vi "Create-Destroy.vi"(8 "Error In":errorcluster) -> (0 "Error Out":errorcluster)   [LabVIEW 2017, in "Tests.lvlib"]
uses:
  Tests.lvlib
  <vilib>/addons/_JKI Toolkits/Caraya/classes/Test/Test.lvclass
  <vilib>/addons/_JKI Toolkits/Caraya/classes/Assert/Assert.lvclass
  src/LabSSH2/Public/Context/Context.lvclass
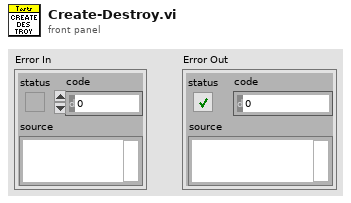
[diagram p1: front panel]
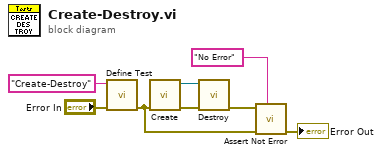
[diagram p0: block diagram]
diagram:
  n1 = call <vilib>:"Define Test.vi"("error in (no error)"="Error In", "Label (VI Title)"="Create-Destroy") -> ("error out"=w4:errorcluster)  [unwired: 9 in]
  n2 = call "Create.vi"("Error In"=w4) -> ("Error Out"=w2:errorcluster, "LabSSH2"=w3:refnum<class "Context.lvclass">)  [unwired: 9 in]
  n3 = call "Destroy.vi"("Error In"=w2, "LabSSH2"=w3) -> ("Error Out"=w1:errorcluster)  [unwired: 9 in]
  n4 = call <vilib>:"Assert Not Error.vi"("Label"="No Error", "error in (no error)"=w4, "Not Error?"=w1) -> ("error out"=→"Error Out":errorcluster)  [unwired: 8 in]
